vi "SO2 43c Serial Data Recording & DECADEv3.6_test.vi"() -> ()   [LabVIEW 2014]
uses:
  <vilib>/Instr/_visa.llb/VISA Set IO Buffer Mask.ctl
  <vilib>/Platform/TimedLoop/XDataNode/timing_clust.ctl
  <vilib>/Platform/TimedLoop/XDataNode/nitl_modes.ctl
  <vilib>/Platform/TimedLoop/XDataNode/wakeup.ctl
  C:/Program Files (x86)/National Instruments/LabVIEW 2014/examples/Data Communication/Network Streams/Simple Network Streams/support/Network Stream Command.ctl
  <vilib>/Utility/error.llb/whitespace.ctl
  <vilib>/Instr/_visa.llb/VISA Configure Serial Port (Instr).vi
  <vilib>/Utility/tcp.llb/UDP Multicast Write-Only Open.vi
  <vilib>/platform/TimedLoop/XDataNode/XDataNode.xnode
  <vilib>/Platform/TimedLoop/XDataNode/XDNodeRunTimeDep.lvlib
panel:
  out "Default file name":string
  out "Stop File Write":bool
  out "error out 4":errorcluster
  out "Data Array UDP":string[](array[string])
  out "Slope":dbl=0.87463
  out "Offset":dbl
  out "Simulate TWA Conc":dbl
  out "8hr_TWA_limit":i32=490
  out "10mins_STEL_limit":i32=700
  out "Simulate STEL Conc":dbl
  out "Simulate\nconc":bool
  out "q_size 2":i32
  out "8hr_so2_avg 2":dbl=1.0
  out "10min_so2_avg":dbl=1.0
  out "q_size":i32
  in  "Clear Display\nErrors":bool
  in  "dummy2":string="0"
  out "Data Processing":bool
  out "Serial Visa Error":errorcluster
  out "SEPTIC TCP Error Out":errorcluster
  out "TCP packet\nSend to SEPTIC":bool
  in  "Time Stamp\nOffset":u32=1
  out "Data Array TCP":string[](array[string])
  out "UDP packet \nstatus":bool
  out "UDP_Out_Error":errorcluster
  out "FISH TCP Error Out":errorcluster
  out "TCP packet\nSend to FISH":bool
  out "TCP Binary Packet":string
  out "Scan from String Error Counter\nfrom process loop":i32
  out "Read Error Counter\nfrom process loop":i32
  in  "milliseconds to wait":u32=330
  in  "ID":string="«"
  in  "VISA resource name":refnum<visa-resource-name>="ASRL6::INSTR"
  out "Data In Array":string[](array[string])
  out "UDP_ASCII_Out":string
  out "UDP_Pack_num":u32
  out "Flight Number":string
  in  "dummy1":string="00"
  out "Data String":string
  out "Internal packet":string[](array[string])
  out "RAW DATA":string
  in  "stop":bool
  out "Number of Send & Read Error\nfrom Acquire Loop":i32
  out "Command In":string
  # "SO2_conc"
  # "PMT_Volt"
  # "Lamp_Volt"
  # "Lamp_Intensity_Hz"
  # "Internal_Temp_degC"
  # "Reaction_Chamber_Temp_degC"
  # "Reaction_Chamber_Press_mmHg"
  # "Sample_Flow_litre_per_minute"
  # "Flag"
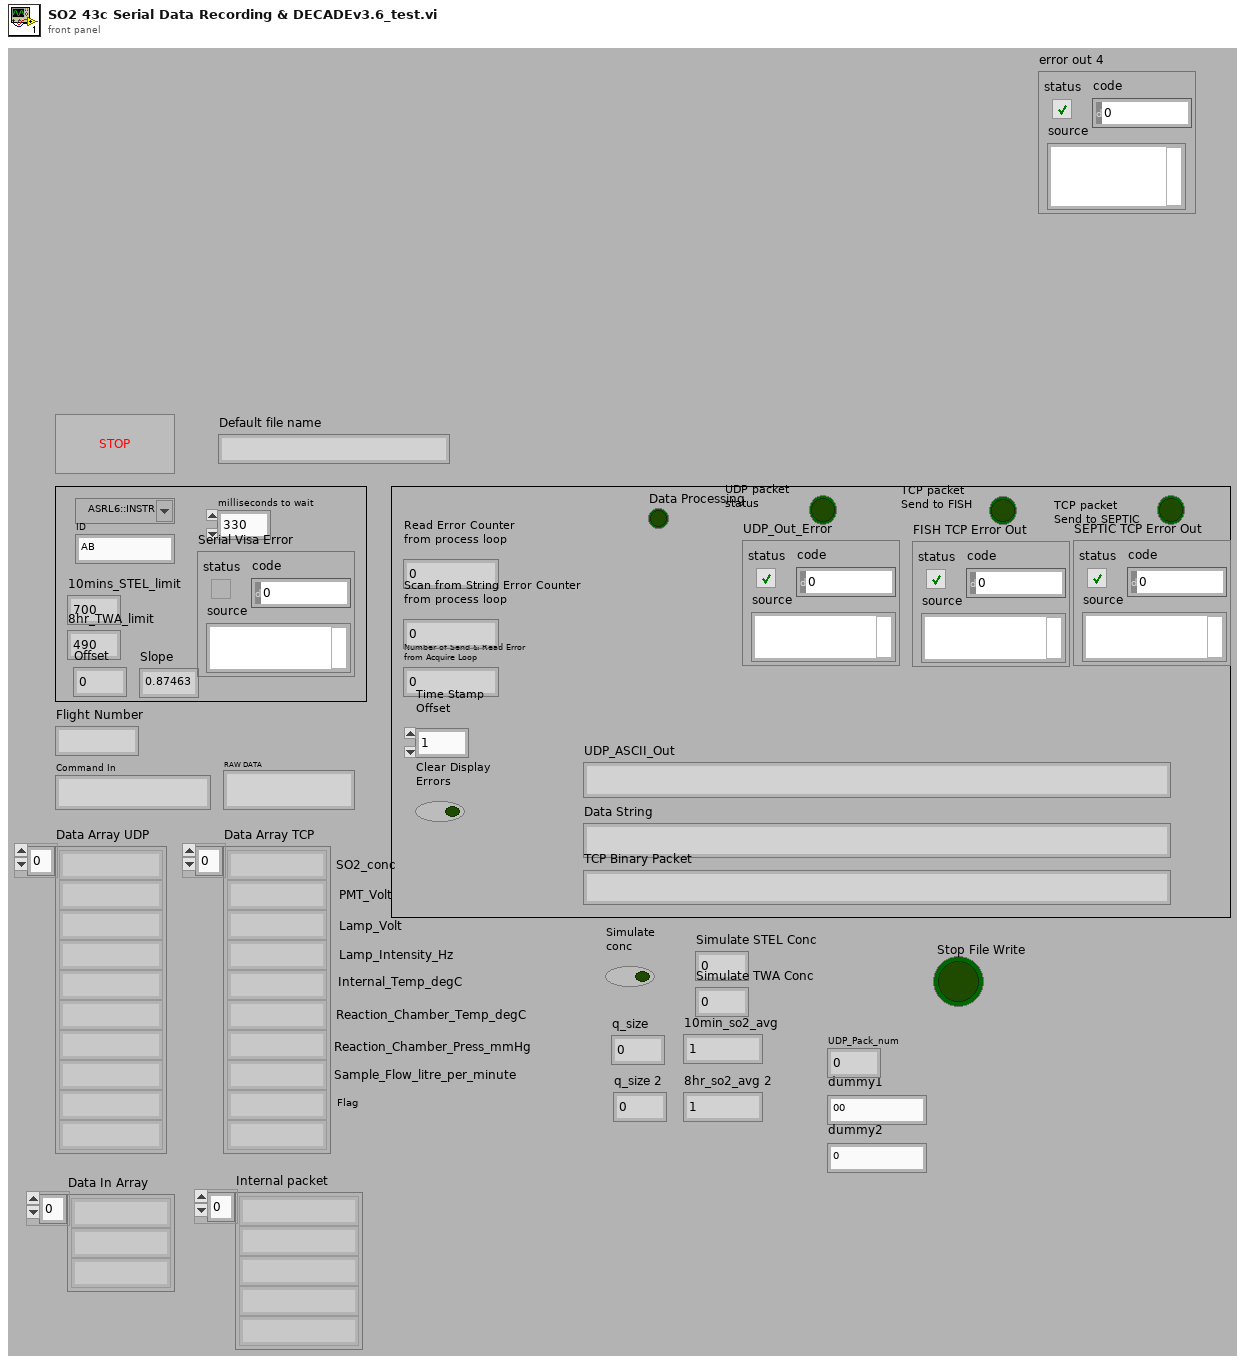
[diagram p1: front panel]
types:
  T1 = typedef "VISA Set IO Buffer Mask.ctl" = u16
  T2 = typedef "Network Stream Command.ctl" = cluster{"Message":string, "Message Data":variant}
  T3 = typedef "XDNodeRunTimeDep.lvlib/timing_clust.ctl" = cluster{"Expected End [f-1]":u64, "Actual End [f-1]":u64, "Finished Late? [f-1]":bool, "Expected End [i-1]":u64, "Actual End [i-1]":u64, "Finished Late? [i-1]":bool, "Expected Start [i]":u64, "Actual Start [i]":u64, "Expected Start [f]":u64, "Actual Start [f]":u64, "Source Name":string, "Structure Name":string, "Period":i64, "Deadline":i64, "Offset":i64, "Start":i64, "Priority":i32, "Timeout":i32, "Mode":T4, "Wakeup Reason":T5, "Error":errorcluster, "Source Type":string, "Secondary Source Type":string, "Global End Time":u64, "Global Start Time":u64, "Frame Duration":u64, "Iteration Duration":u64, "Assigned CPU":i32, "I/O Scan Engine Mode":u32}
  T4 = typedef "XDNodeRunTimeDep.lvlib/nitl_modes.ctl" = enum32{"No Change", "Process missed periods, maintain original phase", "Discard missed periods, maintain original phase", "Process missed periods, ignore original phase", "Discard missed periods, ignore original phase"}
  T5 = typedef "XDNodeRunTimeDep.lvlib/wakeup.ctl" = enum32{"Normal", "Aborted", "Asynchronous wakeup", "Timing source error", "Timed loop error", "Timeout"}
  T6 = enum16{"open", "replace", "create", "open or create", "replace or create", "replace or create with confirmation"}
  T7 = typedef "whitespace.ctl" = u16
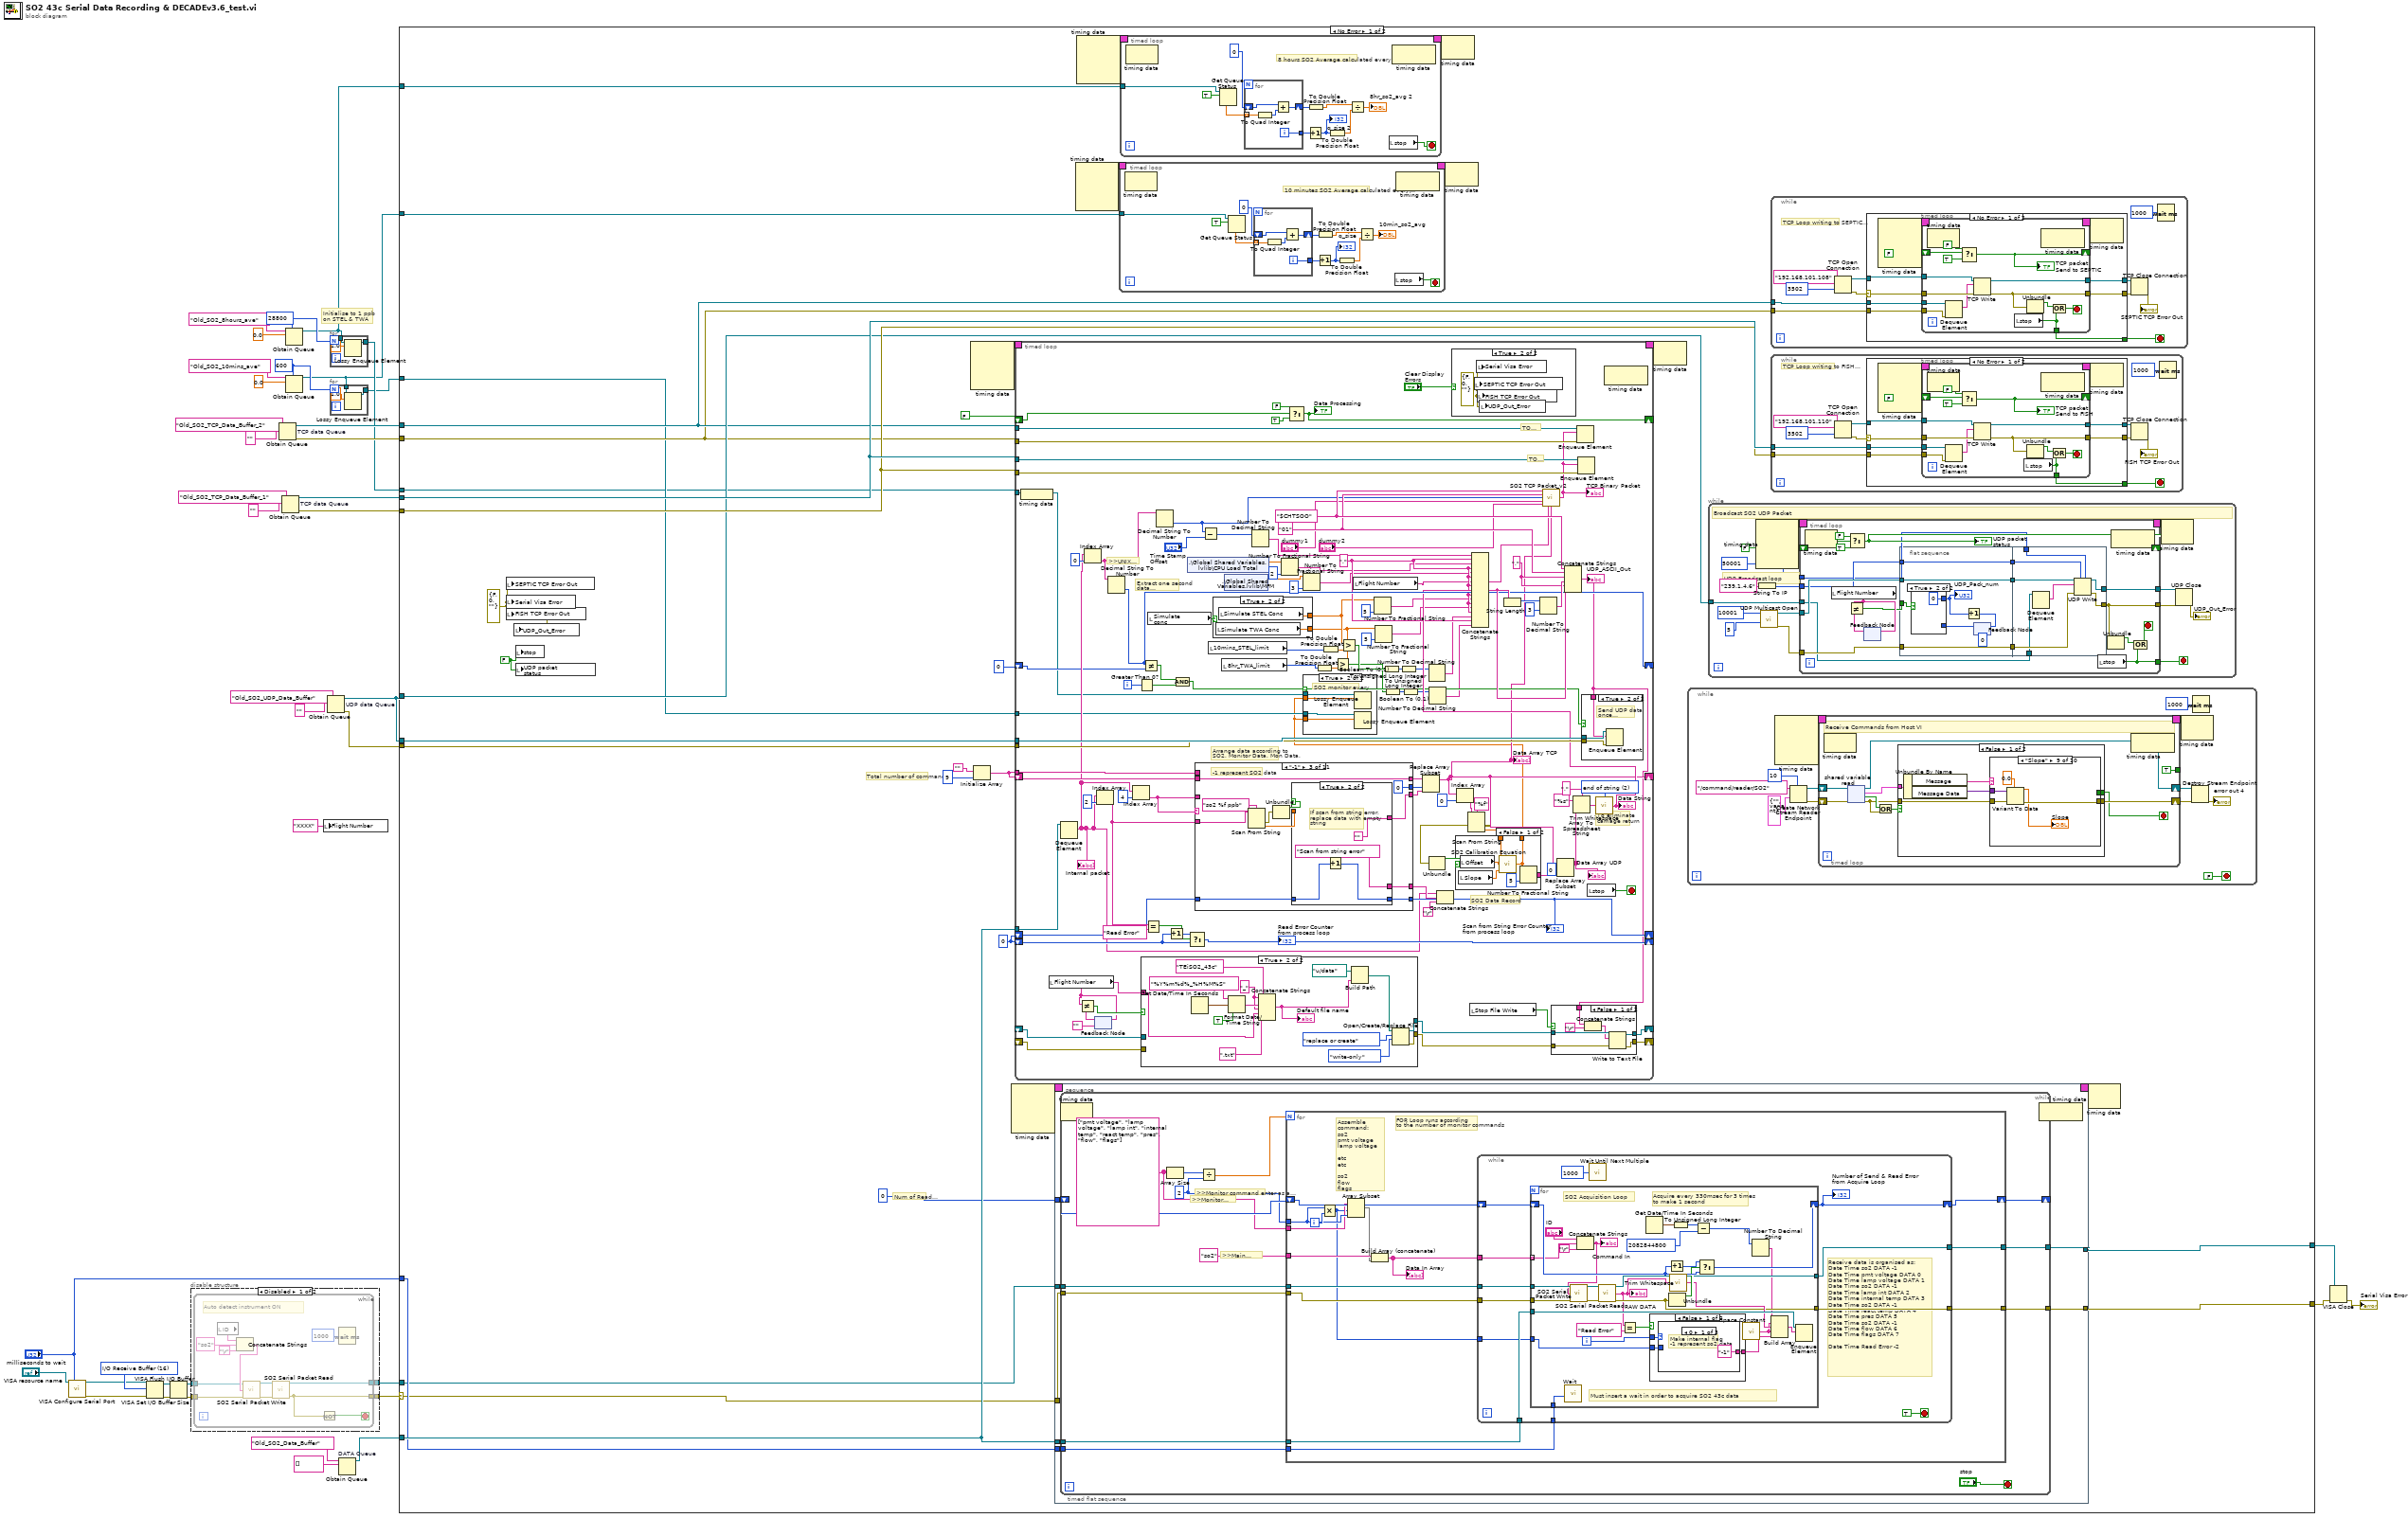
[diagram p0: block diagram]
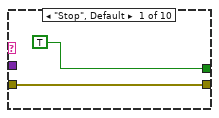
[diagram p3: hidden frame]
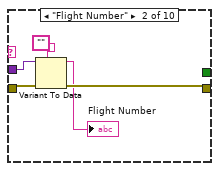
[diagram p4: hidden frame]
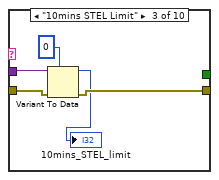
[diagram p5: hidden frame]
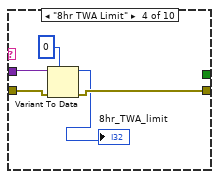
[diagram p6: hidden frame]
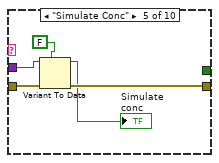
[diagram p7: hidden frame]
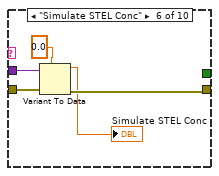
[diagram p8: hidden frame]
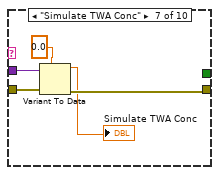
[diagram p9: hidden frame]
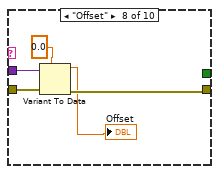
[diagram p10: hidden frame]
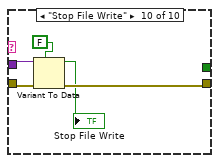
[diagram p11: hidden frame]
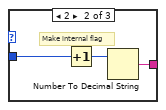
[diagram p13: hidden frame]
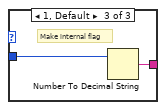
[diagram p14: hidden frame]
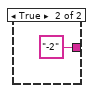
[diagram p15: hidden frame]
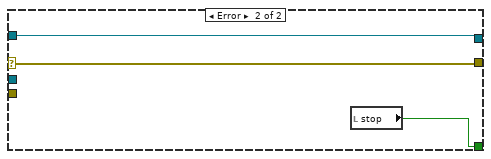
[diagram p16: hidden frame]
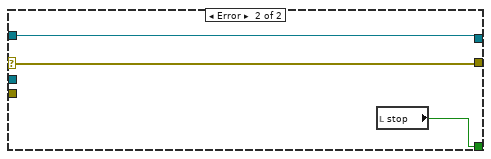
[diagram p18: hidden frame]
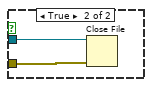
[diagram p20: hidden frame]
diagram:
  w10 = T1 16 items=["I/O Receive Buffer"=16, "I/O Transmit Buffer"=32, "I/O Receive and Transmit Buffer"=48] ("Mask")
  w16 = 28800 ("max queue size (-1, unlimited)")
  w13 = 600 ("max queue size (-1, unlimited)")
  # "Initialise to 1 ppb\non STEL & TWA"
  n1 = call-poly "VISA Configure Serial Port"("VISA resource name"="VISA resource name", "timeout (10sec)"="milliseconds to wait") -> ("VISA resource name out"=w9:refnum<visa-resource-name>, "error out"=w8:errorcluster)  [unwired: 12 in]
  n2 = VISA Set I/O Buffer Size(VISA resource name=w9, mask (16)=w10, error in (no error)=w8) -> (VISA resource name out=w6:refnum<visa-resource-name>, error out=w7:errorcluster)  [unwired: 1 in]
  n3 = VISA Flush I/O Buffer(VISA resource name=w6, error in (no error)=w7) -> (VISA resource name out=w5:refnum<visa-resource-name>, error out=w4:errorcluster)  [unwired: 1 in]
  n4 = disable-structure shown="Disabled" {
    disable-tunnel: w5 -> [w44 _]
    disable-tunnel: w4 -> [w43 _]
    disable-tunnel: [w42 _] -> w3
    disable-tunnel: [w41 _] -> w2
    frame Disabled {
      n5 = while {
        tunnel: w44 -> [w52]
        tunnel: w43 -> [w51]
        tunnel: [w47] -> w42
        tunnel: [w46] -> w41
        stop <- w48 stop-if-true
        # "Auto detect instrument ON"
        n6 = local read "ID"() -> (w55:string)
        n7 = Concatenate Strings(w55, "so2" ("string"), "\r") -> (w53:string)
        n8 = call "SO2 Serial Packet Write.vi"("VISA resource name In"=w52, "Data in"=w53, "error in (no error)"=w51) -> ("VISA resource name Out"=w49:refnum<visa-resource-name>, "error out"=w50:errorcluster)  [unwired: 11 in]
        n9 = call "SO2 Serial Packet Read.vi"("VISA resource In"=w49, "error in"=w50) -> ("VISA resource Out"=w46:refnum<visa-resource-name>, "error out"=w47:errorcluster)  [unwired: 11 in, 1 out]
        n10 = Not(x=w47) -> (.not. x?=w48:bool)
        n11 = Wait (ms)(milliseconds to wait=u32 1000) -> ()  [unwired: 1 out]
      }
    }
    frame Enabled {
    }
  }
  n12 = Obtain Queue "TCP data Queue"(name (unnamed)="Old_SO2_TCP_Data_Buffer_2", element data type="") -> (queue out=w23:refnum<queue>, error out=w22:errorcluster)  [unwired: 3 in, 1 out]
  n13 = Obtain Queue "TCP data Queue"(name (unnamed)="Old_SO2_TCP_Data_Buffer_1", element data type="") -> (queue out=w31:refnum<queue>, error out=w30:errorcluster)  [unwired: 3 in, 1 out]
  n14 = Obtain Queue(max queue size (-1, unlimited)=w16, name (unnamed)="Old_SO2_8hours_ave", element data type=0.0 ("index")) -> (queue out=w15:refnum<queue>)  [unwired: 2 in, 2 out]
  n15 = Obtain Queue(max queue size (-1, unlimited)=w13, name (unnamed)="Old_SO2_10mins_ave", element data type=0.0 ("index")) -> (queue out=w12:refnum<queue>)  [unwired: 2 in, 2 out]
  n16 = local write "Flight Number"("XXXX" ("Flight Number")) -> ()
  n17 = Obtain Queue "UDP data Queue"(name (unnamed)="Old_SO2_UDP_Data_Buffer", element data type="") -> (queue out=w26:refnum<queue>, error out=w27:errorcluster)  [unwired: 3 in, 1 out]
  n18 = for {
    N: w16 -> [_]
    tunnel: w15 -> [w59]
    tunnel: [w58] -> w14
    n19 = Lossy Enqueue Element(queue=w59, element=1.0) -> (queue out=w58:refnum<queue>)  [unwired: 1 in, 3 out]
  }
  n20 = for {
    N: w13 -> [_]
    tunnel: [w62] -> w11
    tunnel: w12 -> [w60]
    n21 = Lossy Enqueue Element(queue=w60, element=1.0) -> (queue out=w62:refnum<queue>)  [unwired: 1 in, 3 out]
  }
  n22 = Obtain Queue "DATA Queue"(name (unnamed)="Old_SO2_Data_Buffer", element data type=string[] []) -> (queue out=w38:refnum<queue>)  [unwired: 3 in, 2 out]
  n23 = case shown="No Error" w3 {
    selector: w3 -> [w65 w822]
    tunnel: [w96 w822] -> w35
    tunnel: [w95 w821] -> w36
    tunnel: w38 -> [w92 _]
    tunnel: w2 -> [w66 w821]
    tunnel: w31 -> [w85 _]
    tunnel: w30 -> [w84 _]
    tunnel: w26 -> [w83 _]
    tunnel: w27 -> [w82 _]
    tunnel: w26 -> [w81 _]
    tunnel: w23 -> [w79 _]
    tunnel: w22 -> [w78 _]
    tunnel: "milliseconds to wait" -> [w77 _]
    tunnel: w12 -> [w74 _]
    tunnel: w15 -> [w73 _]
    tunnel: w11 -> [w72 _]
    tunnel: w14 -> [w71 _]
    frame No Error {
      w75 = errorcluster {"status"=FALSE, "code"=0, "source"=""} ("UDP Error Out")
      w87 = 0
      w86 = FALSE ("stop")
      # "Num of Read Error"
      # "Total number of commands"
      n24 = local write "SEPTIC TCP Error Out"(w75) -> ()
      n25 = local write "Serial Visa Error"(w75) -> ()
      n26 = local write "FISH TCP Error Out"(w75) -> ()
      n27 = local write "UDP_Out_Error"(w75) -> ()
      n28 = local write "stop"(w86) -> ()
      n29 = local write "UDP packet \nstatus"(w86) -> ()
      n30 = node-c288() -> (w94:T3)  [unwired: 4 in]
      n31 = Initialize Array("", 9) -> (w88:string[])
      n32 = node-c288() -> (w64:T3)  [unwired: 4 in]
      n33 = timed-loop {
        timing: w94 -> [_]
        timing-out: [_] -> w93
        tunnel: w92 -> [w568]
        shift-right: [w485] -> _
        shift-left: w88 -> [w558]
        shift-right: [w549] -> _
        shift-left: w87 -> [w546]
        tunnel: w88 -> [w548]
        shift-right: [w544] -> _
        shift-left: w87 -> [w545]
        tunnel: w85 -> [w539]
        tunnel: w84 -> [w538]
        tunnel: w83 -> [w537]
        tunnel: w82 -> [w536]
        shift-right: [w528] -> _
        shift-left: 0 -> [w531]
        tunnel: w79 -> [w527]
        tunnel: w78 -> [w526]
        shift-right: [w517] -> _
        shift-left: FALSE -> [w520]
        tunnel: w72 -> [w511]
        tunnel: w71 -> [w510]
        shift-right: [w470] -> _
        shift-left: _ -> [w467]
        shift-right: [w469] -> _
        shift-left: _ -> [w465]
        i -> [w529]
        stop <- w566 stop-if-true
        w554 = T7 2 items=["both", "start of string", "end of string"] ("location (both)")
        w509 = ","
        w541 = "01"
        w560 = ","
        w542 = "$CHTSOO"
        # "TO SEPTIC"
        # "TO FISH"
        # "Extract one second data\nfor UDP sending"
        # "Arrange data according to\nSO2, Monitor Data, Mon Data,"
        # "To eliminate\ncarriage return"
        # ">>UNIX TIME>>"
        # "SO2 Data Record"
        n34 = node-c288() -> ()  [unwired: 1 in]
        n35 = local read "Flight Number"() -> (w466:string)
        n36 = Dequeue Element(queue=w568) -> (element=w534:string[])  [unwired: 2 in, 3 out]
        "Internal packet" <- w534
        n37 = Index Array(array=w534, index=0) -> (element=w533:string)
        n38 = feedback #1("" ("Flight Number")) -> (w475:string)
        n39 = Not Equal?(x=w466, y=w475) -> (x != y?=w473:bool)
        n40 = feedback-in #1(w466) -> ()
        n41 = Index Array(array=w534, index=2) -> (element=w552:string)
        n42 = Decimal String To Number(string=w533) -> (number=w528:i32)  [unwired: 2 in, 1 out]
        n43 = Index Array(array=w534, index=4) -> (element=w516:string)
        n44 = Greater Than 0?(x=w529) -> (x > 0?=w532:bool)
        n45 = case shown="True" w473 {
          tunnel: [w570 w573] -> w472
          tunnel: [w569 w572] -> w468
          tunnel: w467 -> [w570 _]
          tunnel: w465 -> [w569 _]
          tunnel: w466 -> [_ w571]
          frame False {
          }
          frame True {
            w580 = "_" ("string")
            n46 = Get Date/Time In Seconds() -> (seconds since 1Jan1904=w581:timestamp)
            n47 = Format Date/Time String(time format string (%c)="%Y%m%d%_%H%M%S", seconds (now)=w581, UTC format=TRUE) -> (date/time string=w584:string)
            n48 = Concatenate Strings("TEiSO2_43c" ("string"), w580, w584, w580, w571, ".txt" ("string")) -> (w578:string)
            "Default file name" <- w578
            n49 = Build Path(base path=path "u:/data", name or relative path=w578) -> (appended path=w574:path)
            n50 = Open/Create/Replace File(file path (use dialog)=w574, operation (0:open)=T6."replace or create", access (0:read/write)=enum16{"read/write", "read-only", "write-only"}."write-only") -> (refnum out=w573:refnum<file>, error out=w572:errorcluster)  [unwired: 3 in, 1 out]
          }
        }
        n51 = Not Equal?(x=w528, y=w531) -> (x != y?=w530:bool)
        n52 = Equal?(x=w552, y="Read Error") -> (x = y?=w550:bool)
        n53 = local read "Simulate\nconc"() -> (w479:bool)
        n54 = Decimal String To Number(string=w533) -> (number=w523:i32)  [unwired: 2 in, 1 out]
        n55 = Increment(x=w546) -> (x+1=w547:i32)
        n56 = Compound Arithmetic op=AND(w530, w532) -> (w512:bool)
        n57 = shared-variable ".\\Global Shared Variables.lvlib\\CPU Load Total"() -> (w463:dbl)  [unwired: 1 in, 1 out]
        n58 = Select(t=w547, s=w550, f=w546) -> (s? t:f=w549:i32)
        "Read Error Counter\nfrom process loop" <- w549
        n59 = case shown="\"-1\"" w516 {
          tunnel: w516 -> [w620 _ _ w656 w677 w698 w720 w742 w764 w786 w808]
          tunnel: w558 -> [w621 _ w635 w657 w678 w699 w721 w743 w765 w787 w809]
          tunnel: w552 -> [_ _ w632 w652 w673 w695 w717 w739 w761 w783 w805]
          tunnel: [w621 w624 w635 w657 w678 w699 w721 w743 w765 w787 w809] -> w492
          tunnel: [w618 _ 0 ("index") w654 w675 w696 w718 w740 w762 w784 w806] -> w491
          tunnel: [_ _ w631 w651 w672 w694 w716 w738 w760 w782 w800] -> w557
          tunnel: w548 -> [_ w624 _ _ _ _ _ _ _ _ _]
          tunnel: w545 -> [w616 w623 w628 w648 w669 w689 w712 w733 w756 w777 w799]
          tunnel: [w616 w623 w627 w647 w668 w688 w711 w732 w755 w776 w798] -> w544
          tunnel: ["Internal False Flag Detected" "" w626 w646 w667 w687 w710 w731 w754 w775 w797] -> w543
          frame "False", Default {
            n60 = Decimal String To Number(string=w620) -> (number=w617:i32)  [unwired: 2 in, 1 out]
            n61 = Add(x=w617, y=1) -> (x+y=w618:i32)
          }
          frame "-2" {
            # "Read Error Detected\nMake all data as a space"
          }
          frame "-1" {
            # "-1 represent SO2 data"
            n62 = Scan From String(format string="so2 %f ppb", input string=w632) -> (error out=w630:errorcluster, output 1=w625:dbl)  [unwired: 3 in, 2 out]
            n63 = Unbundle(w630) -> ("status"=w629:bool)  [unwired: 2 out]
            n64 = case shown="True" w629 {
              tunnel: w625 -> [w636 _]
              tunnel: [w640 ""] -> w631
              tunnel: w628 -> [w639 w644]
              tunnel: [w639 w643] -> w627
              tunnel: ["" "Scan from string error"] -> w626
              frame False {
                # "Extract the concentration\nvalue & fixed format"
                n65 = Number To Fractional String(number=w636, precision (6)=i16 5) -> (F-format string=w640:string)  [unwired: 2 in]
              }
              frame True {
                # "If scan from string error,\nreplace data with empty\nstring"
                n66 = Increment(x=w644) -> (x+1=w643:i32)
              }
            }
          }
          frame "0" {
            # "0 represents pmt voltage -0510 volts"
            n67 = Scan From String(format string="pmt voltage %d volts", input string=w652) -> (error out=w650:errorcluster, output 1=w645:i32)  [unwired: 3 in, 2 out]
            n68 = Decimal String To Number(string=w656) -> (number=w655:i32)  [unwired: 2 in, 1 out]
            n69 = Unbundle(w650) -> ("status"=w649:bool)  [unwired: 2 out]
            n70 = case shown="False" w649 {
              tunnel: w645 -> [w661 _]
              tunnel: [w658 w662] -> w651
              tunnel: w648 -> [w660 w665]
              tunnel: [w660 w664] -> w647
              tunnel: ["" "Scan from string error"] -> w646
              tunnel: [w658 w662] -> _
              frame False {
                # "Extract the actual value\n& fixed format"
                n71 = Number To Decimal String(number=w661) -> (decimal integer string=w658:string)  [unwired: 1 in]
              }
              frame True {
                w662 = ""
                # "If scan from string error,\nreplace data with empty\nstring"
                n72 = Increment(x=w665) -> (x+1=w664:i32)
              }
            }
            n73 = Increment(x=w655) -> (x+1=w654:i32)
          }
          frame "1" {
            # "1 represents lamp voltage; lamp voltage 810 volts"
            n74 = Scan From String(format string="lamp voltage %d volts", input string=w673) -> (error out=w671:errorcluster, output 1=w666:i32)  [unwired: 3 in, 2 out]
            n75 = Decimal String To Number(string=w677) -> (number=w676:i32)  [unwired: 2 in, 1 out]
            n76 = Unbundle(w671) -> ("status"=w670:bool)  [unwired: 2 out]
            n77 = case shown="True" w670 {
              tunnel: w666 -> [w682 _]
              tunnel: [w679 w683] -> w672
              tunnel: w669 -> [w681 w686]
              tunnel: [w681 w685] -> w668
              tunnel: ["" "Scan from string error"] -> w667
              tunnel: [w679 w683] -> _
              frame False {
                # "Extract the actual value\n& fixed format"
                n78 = Number To Decimal String(number=w682) -> (decimal integer string=w679:string)  [unwired: 1 in]
              }
              frame True {
                w683 = ""
                # "If scan from string error,\nreplace data with empty\nstring"
                n79 = Increment(x=w686) -> (x+1=w685:i32)
              }
            }
            n80 = Increment(x=w676) -> (x+1=w675:i32)
          }
          frame "2" {
            # "2 represents lamp intensity; lamp int 35867 Hz"
            n81 = Scan From String(format string="lamp int %d Hz", input string=w695) -> (error out=w691:errorcluster, output 1=w692:i32)  [unwired: 3 in, 2 out]
            n82 = Decimal String To Number(string=w698) -> (number=w697:i32)  [unwired: 2 in, 1 out]
            n83 = Unbundle(w691) -> ("status"=w690:bool)  [unwired: 2 out]
            n84 = case shown="True" w690 {
              tunnel: [w700 w705] -> w694
              tunnel: w692 -> [w704 _]
              tunnel: w689 -> [w703 w708]
              tunnel: [w703 w707] -> w688
              tunnel: ["" "Scan from string error"] -> w687
              tunnel: [w700 w705] -> _
              frame False {
                # "Extract the actual value\n& fixed format"
                n85 = Number To Fractional String(number=w704, precision (6)=i16 0) -> (F-format string=w700:string)  [unwired: 2 in]
              }
              frame True {
                w705 = ""
                # "If scan from string error,\nreplace data with empty\nstring"
                n86 = Increment(x=w708) -> (x+1=w707:i32)
              }
            }
            n87 = Increment(x=w697) -> (x+1=w696:i32)
          }
          frame "3" {
            # "3 represents internal temp; internal temp 027.2 deg C, actual 027.2"
            n88 = Scan From String(format string="%[^,], %s %f", input string=w717) -> (error out=w714:errorcluster, output 3=w709:dbl)  [unwired: 7 in, 2 out]
            n89 = Decimal String To Number(string=w720) -> (number=w719:i32)  [unwired: 2 in, 1 out]
            n90 = Unbundle(w714) -> ("status"=w713:bool)  [unwired: 2 out]
            n91 = case shown="True" w713 {
              tunnel: [w722 w727] -> w716
              tunnel: w709 -> [w726 _]
              tunnel: w712 -> [w725 w730]
              tunnel: [w725 w729] -> w711
              tunnel: ["" "Scan from string error"] -> w710
              tunnel: [w722 w727] -> _
              frame False {
                # "Extract the actual value\n& fixed format"
                n92 = Number To Fractional String(number=w726, precision (6)=i16 1) -> (F-format string=w722:string)  [unwired: 2 in]
              }
              frame True {
                w727 = ""
                # "If scan from string error,\nreplace data with empty\nstring"
                n93 = Increment(x=w730) -> (x+1=w729:i32)
              }
            }
            n94 = Increment(x=w719) -> (x+1=w718:i32)
          }
          frame "4" {
            # "4 represents react temp; react temp 045.2 deg C"
            n95 = Scan From String(format string="react temp %f deg C", input string=w739) -> (error out=w735:errorcluster, output 1=w736:dbl)  [unwired: 3 in, 2 out]
            n96 = Decimal String To Number(string=w742) -> (number=w741:i32)  [unwired: 2 in, 1 out]
            n97 = Unbundle(w735) -> ("status"=w734:bool)  [unwired: 2 out]
            n98 = case shown="False" w734 {
              tunnel: [w744 w749] -> w738
              tunnel: w736 -> [w748 _]
              tunnel: w733 -> [w747 w752]
              tunnel: [w747 w751] -> w732
              tunnel: ["" "Scan from string error"] -> w731
              tunnel: [w744 w749] -> _
              frame False {
                # "Extract the actual value\n& fixed format"
                n99 = Number To Fractional String(number=w748, precision (6)=i16 1) -> (F-format string=w744:string)  [unwired: 2 in]
              }
              frame True {
                w749 = ""
                # "If scan from string error,\nreplace data with empty\nstring"
                n100 = Increment(x=w752) -> (x+1=w751:i32)
              }
            }
            n101 = Increment(x=w741) -> (x+1=w740:i32)
          }
          frame "5" {
            # "5 represents chamber pressure; pres 760.0 mm Hg, actual 753.4"
            n102 = Scan From String(format string="%[^,], %s %f", input string=w761) -> (error out=w758:errorcluster, output 3=w753:dbl)  [unwired: 7 in, 2 out]
            n103 = Decimal String To Number(string=w764) -> (number=w763:i32)  [unwired: 2 in, 1 out]
            n104 = Unbundle(w758) -> ("status"=w757:bool)  [unwired: 2 out]
            n105 = case shown="False" w757 {
              tunnel: [w766 w771] -> w760
              tunnel: w753 -> [w770 _]
              tunnel: w756 -> [w769 w774]
              tunnel: [w769 w773] -> w755
              tunnel: ["" "Scan from string error"] -> w754
              tunnel: [w766 w771] -> _
              frame False {
                # "Extract the actual value\n& fixed format"
                n106 = Number To Fractional String(number=w770, precision (6)=i16 1) -> (F-format string=w766:string)  [unwired: 2 in]
              }
              frame True {
                w771 = ""
                # "If scan from string error,\nreplace data with empty\nstring"
                n107 = Increment(x=w774) -> (x+1=w773:i32)
              }
            }
            n108 = Increment(x=w763) -> (x+1=w762:i32)
          }
          frame "6" {
            # "6 represents flow data; flow 0.503 l/m"
            n109 = Scan From String(format string="flow %f l/m", input string=w783) -> (error out=w779:errorcluster, output 1=w780:dbl)  [unwired: 3 in, 2 out]
            n110 = Decimal String To Number(string=w786) -> (number=w785:i32)  [unwired: 2 in, 1 out]
            n111 = Unbundle(w779) -> ("status"=w778:bool)  [unwired: 2 out]
            n112 = case shown="True" w778 {
              tunnel: [w792 ""] -> w782
              tunnel: w780 -> [w791 _]
              tunnel: w777 -> [w790 w795]
              tunnel: [w790 w794] -> w776
              tunnel: ["" "Scan from string error"] -> w775
              frame False {
                # "Extract the actual value\n& fixed format"
                n113 = Number To Fractional String(number=w791, precision (6)=i16 3) -> (F-format string=w792:string)  [unwired: 2 in]
              }
              frame True {
                # "If scan from string error,\nreplace data with empty\nstring"
                n114 = Increment(x=w795) -> (x+1=w794:i32)
              }
            }
            n115 = Increment(x=w785) -> (x+1=w784:i32)
          }
          frame "7" {
            # "7 represents flags data; flags 1c100000"
            n116 = Scan From String(format string="flags %s", input string=w805) -> (error out=w803:errorcluster, output 1=w801:string)  [unwired: 3 in, 2 out]
            n117 = Decimal String To Number(string=w808) -> (number=w807:i32)  [unwired: 2 in, 1 out]
            n118 = Unbundle(w803) -> ("status"=w802:bool)  [unwired: 2 out]
            n119 = case shown="False" w802 {
              tunnel: w801 -> [w812 _]
              tunnel: [w812 ""] -> w800
              tunnel: w799 -> [w811 w815]
              tunnel: [w811 w814] -> w798
              tunnel: ["" "Scan from string error"] -> w797
              frame False {
                # "Extract the actual value\n& fixed format"
              }
              frame True {
                # "If scan from string error,\nreplace data with empty\nstring"
                n120 = Increment(x=w815) -> (x+1=w814:i32)
              }
            }
            n121 = Increment(x=w807) -> (x+1=w806:i32)
          }
        }
        "Scan from String Error Counter\nfrom process loop" <- w544
        n122 = Subtract(x=w523, y="Time Stamp\nOffset") -> (x-y=w524:u32)
        n123 = local read "10mins_STEL_limit"() -> (w477:i32)
        n124 = case shown="True" w479 {
          tunnel: [w604 w606] -> w505
          tunnel: [w603 w605] -> w503
          frame False {
            n125 = local read "10min_so2_avg"() -> (w604:dbl)
            n126 = local read "8hr_so2_avg 2"() -> (w603:dbl)
          }
          frame True {
            n127 = local read "Simulate TWA Conc"() -> (w605:dbl)
            n128 = local read "Simulate STEL Conc"() -> (w606:dbl)
          }
        }
        n129 = local read "8hr_TWA_limit"() -> (w476:i32)
        n130 = shared-variable ".\\Global Shared Variables.lvlib\\MFM"() -> (w461:dbl)  [unwired: 1 in, 1 out]
        n131 = Number To Decimal String(number=w524) -> (decimal integer string=w521:string)  [unwired: 1 in]
        n132 = Number To Fractional String(number=w463, precision (6)=i16 2) -> (F-format string=w459:string)  [unwired: 2 in]
        n133 = Select(t=FALSE, s=w520, f=TRUE) -> (s? t:f=w517:bool)
        "Data Processing" <- w517
        n134 = Number To Fractional String(number=w461, precision (6)=i16 3) -> (F-format string=w458:string)  [unwired: 2 in]
        n135 = To Double Precision Float(number=w476) -> (double precision float=w506:dbl)
        n136 = To Double Precision Float(number=w477) -> (double precision float=w507:dbl)
        n137 = Greater?(x=w503, y=w506) -> (0:w496:bool)
        n138 = Greater?(x=w505, y=w507) -> (0:w498:bool)
        n139 = local read "Flight Number"() -> (w478:string)
        n140 = Number To Fractional String(number=w505, precision (6)=i16 5) -> (F-format string=w502:string)  [unwired: 2 in]
        n141 = Number To Fractional String(number=w503, precision (6)=i16 5) -> (F-format string=w501:string)  [unwired: 2 in]
        n142 = Boolean To (0,1)(Boolean=w498) -> (0, 1=w500:i16)
        n143 = Boolean To (0,1)(Boolean=w496) -> (0, 1=w499:i16)
        n144 = To Unsigned Long Integer(number=w500) -> (unsigned 32bit integer=w494:u32)
        n145 = To Unsigned Long Integer(number=w499) -> (unsigned 32bit integer=w493:u32)
        n146 = Replace Array Subset(array=w492, new element=w557, index=w491) -> (w485:string[])
        "Data Array TCP" <- w485
        n147 = Number To Decimal String(number=w494) -> (decimal integer string=w497:string)  [unwired: 1 in]
        n148 = Number To Decimal String(number=w493) -> (decimal integer string=w495:string)  [unwired: 1 in]
        n149 = Concatenate Strings(w534, w543, "\r") -> ()  [unwired: 1 out]
        n150 = case shown="True" "Clear Display\nErrors" {
          frame False {
          }
          frame True {
            w611 = errorcluster {"status"=FALSE, "code"=0, "source"=""} ("UDP Error Out")
            n151 = local write "SEPTIC TCP Error Out"(w611) -> ()
            n152 = local write "Serial Visa Error"(w611) -> ()
            n153 = local write "FISH TCP Error Out"(w611) -> ()
            n154 = local write "UDP_Out_Error"(w611) -> ()
          }
        }
        n155 = Index Array(array=w485, index=0) -> (element=w489:string)
        n156 = Scan From String(format string="%f", input string=w489) -> (error out=w481:errorcluster, output 1=w487:dbl)  [unwired: 3 in, 2 out]
        n157 = Unbundle(w481) -> ("status"=w480:bool)  [unwired: 2 out]
        n158 = case shown="False" w480 {
          tunnel: w487 -> [w599 _]
          tunnel: [w598 ""] -> w486
          tunnel: [w597 0.0 ("Output")] -> w482
          frame False {
            n159 = local read "Slope"() -> (w595:dbl)
            n160 = local read "Offset"() -> (w596:dbl)
            n161 = call "SO2 Calibration Equation.vi"("Input"=w599, "Offset"=w596, "Slope"=w595) -> ("Output"=w597:dbl)  [unwired: 12 in]
            n162 = Number To Fractional String(number=w597, precision (6)=i16 5) -> (F-format string=w598:string)  [unwired: 2 in]
          }
          frame True {
          }
        }
        n163 = case shown="True" w512 {
          tunnel: w511 -> [_ w610]
          tunnel: w482 -> [_ w607]
          tunnel: w482 -> [_ w609]
          tunnel: w510 -> [_ w608]
          frame False {
          }
          frame True {
            # "SO2 monitor every second"
            n164 = Lossy Enqueue Element(queue=w610, element=w607) -> ()  [unwired: 1 in, 4 out]
            n165 = Lossy Enqueue Element(queue=w608, element=w609) -> ()  [unwired: 1 in, 4 out]
          }
        }
        n166 = local read "Stop File Write"() -> (w471:bool)
        n167 = call "SO2 TCP Packet_v2.vi"("ID"=w542, "Version"=w541, "utc_time"=w523, "dummy1"="dummy1", "dummy2"="dummy2", "Flight Number"=w478, "Data Array"=w485) -> ("TCP Binary Packet"=w525:string)  [unwired: 8 in]
        "TCP Binary Packet" <- w525
        n168 = Replace Array Subset(array=w485, new element=w486, index=0) -> (w484:string[])
        "Data Array UDP" <- w484
        n169 = Array To Spreadsheet String(delimiter (Tab)=",", array=w484, 3:"%s" ("format string")) -> (spreadsheet string=w553:string)
        n170 = Enqueue Element(queue=w527, element=w525, error in (no error)=w526) -> ()  [unwired: 1 in, 3 out]
        n171 = Enqueue Element(queue=w539, element=w525, error in (no error)=w538) -> ()  [unwired: 1 in, 3 out]
        n172 = local read "stop"() -> (w566:bool)
        n173 = call <vilib>:"Trim Whitespace.vi"("string"=w553, "location (both)"=w554) -> ("trimmed string"=w515:string)
        "Data String" <- w515
        n174 = Concatenate Strings(w521, w509, w459, w509, w458, w509, w478, w509, w515, w509, w502, w509, w501, w509, w497, w509, w495) -> (w559:string)
        n175 = String Length(string=w559) -> (length=w563:i32)
        n176 = Number To Decimal String(number=w563, width (-)=i16 3) -> (decimal integer string=w561:string)
        n177 = Concatenate Strings(w542, w541, w560, w561, w560, w559) -> (w464:string)
        "UDP_ASCII_Out" <- w464
        n178 = case shown="False" w471 {
          tunnel: w464 -> [w590 _]
          tunnel: w472 -> [w592 w594]
          tunnel: w468 -> [w591 w593]
          tunnel: [w587 _] -> w470
          tunnel: [w586 _] -> w469
          frame False {
            n179 = Concatenate Strings(w590, "\r") -> (w588:string)
            n180 = Write to Text File(file (use dialog)=w592, text=w588, error in=w591) -> (refnum out=w587:refnum<file>, error out=w586:errorcluster)  [unwired: 2 out]
          }
          frame True {
            n181 = Close File(refnum=w594, error in=w593) -> ()  [unwired: 2 out]
          }
        }
        n182 = case shown="True" w512 {
          tunnel: w537 -> [_ w614]
          tunnel: w536 -> [_ w613]
          tunnel: w464 -> [_ w612]
          frame False {
          }
          frame True {
            # "Send UDP data once\na second"
            n183 = Enqueue Element(queue=w614, element=w612, error in (no error)=w613) -> ()  [unwired: 1 in, 3 out]
          }
        }
        n184 = node-c288() -> ()  [unwired: 1 in, 1 out]
      }
      n185 = timed-sequence {
        timing: w64 -> [_]
        timing-out: [_] -> w63
        tunnel: [w184] -> w96
        tunnel: [w183] -> w95
        tunnel: w92 -> [w182]
        tunnel: 0 -> [w181]
        tunnel: w77 -> [w180]
        tunnel: w66 -> [w179]
        tunnel: w65 -> [w178]
        n186 = timed-flat-sequence {
          tunnel: [w191] -> w184
          tunnel: [w190] -> w183
          tunnel: w182 -> [w189]
          tunnel: w181 -> [w188]
          tunnel: w180 -> [w187]
          tunnel: w179 -> [w186]
          tunnel: w178 -> [w185]
          n187 = node-c288() -> ()  [unwired: 1 in, 1 out]
          n188 = while {
            tunnel: [w194] -> w191
            tunnel: w186 -> [w205]
            tunnel: w185 -> [w204]
            tunnel: [w203] -> w190
            tunnel: w189 -> [w202]
            shift-right: [w200] -> _
            shift-left: w188 -> [w201]
            tunnel: w187 -> [w192]
            stop <- "stop" stop-if-true
            w195 = 2
            w197 = string[] ["pmt voltage", "lamp voltage", "lamp int", "internal temp", "react temp", "pres", "flow", "flags"]
            # ">>Monitor command enter as a pair>>"
            # ">>Main commands>>"
            # ">>Monitor Command>>"
            n189 = Array Size(array=w197) -> (size(s)=w198:i32)
            n190 = Divide(x=w198, y=w195) -> (x/y=w196:dbl)
            n191 = for {
              N: w196 -> [_]
              tunnel: w205 -> [w213]
              tunnel: w204 -> [w212]
              tunnel: [w220] -> w194
              shift-right: [w218] -> w200
              shift-left: w201 -> [w219]
              tunnel: [w217] -> w203
              tunnel: w202 -> [w216]
              tunnel: w197 -> [w209]
              tunnel: "so2" -> [w214]
              tunnel: w195 -> [w210]
              tunnel: w192 -> [w206]
              i -> [w211]
              # "FOR Loop runs according\nto the number of monitor commands"
              # "Assemble command:\nso2\npmt voltage\nlamp voltage\n\netc\netc\n\nso2\nflow\nflags"
              n192 = Multiply(x=w210, y=w211) -> (x*y=w207:i32)
              n193 = Array Subset(array=w209, index=w207, length=w210) -> (w208:string[])
              n194 = Build Array (concatenate)(w214, w208) -> (w215:string[])
              "Data In Array" <- w215
              n195 = while {
                tunnel: [w232] -> w220
                tunnel: w215 -> [w230]
                tunnel: [w228] -> w217
                tunnel: w216 -> [w227]
                tunnel: w212 -> [w226]
                tunnel: w213 -> [w225]
                tunnel: w207 -> [w224]
                shift-right: [w229] -> w218
                shift-left: w219 -> [w231]
                tunnel: w206 -> [w221]
                stop <- TRUE stop-if-true
                # "Receive data is organised as:\nDate Time so2 DATA -1\nDate Time pmt voltage DATA 0\nDate Time lamp voltage DATA 1\nDate Time so2 DATA -1\nDate Time lamp int DATA 2\nDate Time internal temp DATA 3\nDate Time so2 DATA -1\nDate Time react temp DATA 4\nDate Time pres DATA 5\nDate Time so2 DATA -1\nDate Time flow DATA 6\nDate Time flags DATA 7\n\nDate Time Read Error -2"
                n196 = for {
                  tunnel: w226 -> [w249]
                  tunnel: [w250] -> w232
                  tunnel: w230 -> [w247] mode=indexing
                  tunnel: [w251] -> w228
                  tunnel: w227 -> [w257]
                  tunnel: w225 -> [w252]
                  tunnel: w224 -> [w246]
                  shift-right: [w261] -> w229
                  shift-left: w231 -> [w262]
                  tunnel: w221 -> [w235]
                  i -> [w239]
                  # "Must insert a wait in order to acquire SO2 43c data"
                  # "Acquire every 330msec for 3 times\nto make 1 second"
                  # "SO2 Acquisition Loop"
                  n197 = call "Wait"("Count(mSec)"=w235) -> ()  [unwired: 1 out]
                  n198 = Concatenate Strings("ID", w247, "\r") -> (w245:string)
                  "Command In" <- w245
                  n199 = call "SO2 Serial Packet Write.vi"("VISA resource name In"=w252, "Data in"=w245, "error in (no error)"=w249) -> ("VISA resource name Out"=w254:refnum<visa-resource-name>, "error out"=w253:errorcluster)  [unwired: 11 in]
                  n200 = call "SO2 Serial Packet Read.vi"("VISA resource In"=w254, "error in"=w253) -> ("VISA resource Out"=w251:refnum<visa-resource-name>, "Data Out"=w242:string, "error out"=w250:errorcluster)  [unwired: 11 in]
                  "RAW DATA" <- w242
                  n201 = Equal?(x=w242, y="Read Error") -> (x = y?=w240:bool)
                  n202 = Get Date/Time In Seconds() -> (seconds since 1Jan1904=w234:timestamp)
                  n203 = case shown="False" w240 {
                    tunnel: [w265 "-2"] -> w255
                    tunnel: w239 -> [w264 _]
                    tunnel: w246 -> [w263 _]
                    frame False {
                      n204 = case shown="0" w264 {
                        tunnel: ["-1" w269 w271] -> w265
                        tunnel: w263 -> [_ w267 w270]
                        frame 0 {
                          # "Make internal flag\n-1 represent so2 data"
                        }
                        frame 2 {
                          # "Make internal flag"
                          n205 = Increment(x=w267) -> (x+1=w268:i32)
                          n206 = Number To Decimal String(number=w268) -> (decimal integer string=w269:string)  [unwired: 1 in]
                        }
                        frame 1, Default {
                          # "Make internal flag"
                          n207 = Number To Decimal String(number=w270) -> (decimal integer string=w271:string)  [unwired: 1 in]
                        }
                      }
                    }
                    frame True {
                    }
                  }
                  n208 = Increment(x=w262) -> (x+1=w258:i32)
                  n209 = Unbundle(w250) -> ("status"=w259:bool)  [unwired: 2 out]
                  n210 = call <vilib>:"Trim Whitespace.vi"("string"=w242) -> ("trimmed string"=w256:string)  [unwired: 1 in]
                  n211 = To Unsigned Long Integer(number=w234) -> (unsigned 32bit integer=w238:u32)
                  n212 = Subtract(x=w238, y=u32 2082844800) -> (x-y=w233:u32)
                  n213 = Select(t=w258, s=w259, f=w262) -> (s? t:f=w261:i32)
                  n214 = call <vilib>:"Space Constant.vi"() -> ("String"=w243:string)
                  n215 = Number To Decimal String(number=w233) -> (decimal integer string=w236:string)  [unwired: 1 in]
                  n216 = Build Array(w236, w243, w256, w243, w255) -> (w244:string[])
                  n217 = Enqueue Element(queue=w257, element=w244) -> ()  [unwired: 2 in, 3 out]
                }
                "Number of Send & Read Error\nfrom Acquire Loop" <- w229
                n218 = call "Wait Until Next Multiple"("Count(mSec)"=u32 1000) -> ()  [unwired: 1 out]
              }
            }
          }
          n219 = node-c288() -> ()  [unwired: 1 in, 1 out]
        }
      }
      n220 = node-c288() -> (w68:T3)  [unwired: 4 in]
      n221 = node-c288() -> (w70:T3)  [unwired: 4 in]
      n222 = timed-loop {
        tunnel: w74 -> [w286]
        timing: w68 -> [_]
        timing-out: [_] -> w67
        stop <- w287 stop-if-true
        # "10 minutes SO2 Average calculated every second"
        n223 = node-c288() -> ()  [unwired: 1 in, 1 out]
        n224 = Get Queue Status(queue=w286, return elements? (F)=TRUE) -> (elements=w277:dbl[])  [unwired: 1 in, 7 out]
        n225 = for {
          tunnel: w277 -> [w290] mode=indexing
          tunnel: [w294] -> w283
          shift-right: [w293] -> w281
          shift-left: i64 0 -> [w292]
          i -> [w294]
          n226 = To Quad Integer(1:w290) -> (0:w291:i64)
          n227 = Add(x=w292, y=w291) -> (x+y=w293:i64)
        }
        n228 = Increment(x=w283) -> (x+1=w278:i32)
        "q_size" <- w278
        n229 = To Double Precision Float(number=w281) -> (double precision float=w279:dbl)
        n230 = To Double Precision Float(number=w278) -> (double precision float=w280:dbl)
        n231 = Divide(x=w279, y=w280) -> (x/y=→"10min_so2_avg":dbl)
        n232 = local read "stop"() -> (w287:bool)
        n233 = node-c288() -> ()  [unwired: 1 in, 1 out]
      }
      n234 = timed-loop {
        tunnel: w73 -> [w306]
        timing: w70 -> [_]
        timing-out: [_] -> w69
        stop <- w307 stop-if-true
        # "8 hours SO2 Average calculated every second"
        n235 = node-c288() -> ()  [unwired: 1 in, 1 out]
        n236 = Get Queue Status(queue=w306, return elements? (F)=TRUE) -> (elements=w303:dbl[])  [unwired: 1 in, 7 out]
        n237 = for {
          tunnel: w303 -> [w310] mode=indexing
          tunnel: [w314] -> w302
          shift-right: [w313] -> w300
          shift-left: i64 0 -> [w312]
          i -> [w314]
          n238 = To Quad Integer(1:w310) -> (0:w311:i64)
          n239 = Add(x=w312, y=w311) -> (x+y=w313:i64)
        }
        n240 = Increment(x=w302) -> (x+1=w297:i32)
        "q_size 2" <- w297
        n241 = To Double Precision Float(number=w300) -> (double precision float=w298:dbl)
        n242 = To Double Precision Float(number=w297) -> (double precision float=w299:dbl)
        n243 = Divide(x=w298, y=w299) -> (x/y=→"8hr_so2_avg 2":dbl)
        n244 = local read "stop"() -> (w307:bool)
        n245 = node-c288() -> ()  [unwired: 1 in, 1 out]
      }
      n246 = node-c288(w69) -> ()  [unwired: 1 out]
      n247 = node-c288(w67) -> ()  [unwired: 1 out]
      n248 = node-c288(w93) -> ()  [unwired: 1 out]
      n249 = while {
        stop <- FALSE stop-if-true
        n250 = node-c288() -> (w98:T3)  [unwired: 4 in]
        n251 = Create Network Stream Reader Endpoint(7:10 ("reader buffer size"), 9:T2 {"Message"="", "Message Data"=variant} ("Message Cluster"), 11:"/command/reader/SO2" ("reader url")) -> (0:w104:errorcluster, 3:w105:refnum<k21>)  [unwired: 4 in]
        n252 = timed-loop "Host->Target Command Reader" {
          shift-right: [w115] -> w102
          shift-left: w104 -> [w118]
          shift-right: [w116] -> w101
          shift-left: w105 -> [w117]
          tunnel: [TRUE] -> _
          timing: w98 -> [_]
          timing-out: [_] -> w97
          stop <- w109 stop-if-true
          # "Receive Commands from Host VI"
          n253 = node-c288() -> ()  [unwired: 1 in, 1 out]
          n254 = shared-variable-read(w117, w118) -> (w116:refnum<k21>, w111:errorcluster, w113:bool, w114:T2)  [unwired: 1 in]
          n255 = Or(x=w113, y=w111) -> (x .or. y?=w112:bool)
          n256 = case shown="False" w112 {
            selector: w112 -> [_ w174]
            tunnel: w111 -> [w126 w175]
            tunnel: [w125 w175] -> w115
            tunnel: w114 -> [w123 _]
            tunnel: [w124 w174] -> w109
            frame False {
              n257 = Unbundle By Name(w123) -> ("Message"=w122:string, "Message Data"=w121:variant)
              n258 = case shown="\"Slope\"" w122 {
                tunnel: w126 -> [w128 w133 w138 w143 w148 w152 w157 w162 w167 w173]
                tunnel: [w128 w130 w136 w141 w147 w150 w155 w160 w165 w170] -> w125
                tunnel: w121 -> [_ w132 w137 w142 w146 w153 w158 w163 w168 w172]
                tunnel: [TRUE _ _ _ _ _ _ _ _ _] -> w124
                frame "Stop", Default {
                }
                frame "Flight Number" {
                  n259 = Variant To Data(error in=w133, type="", Variant=w132) -> (data=→"Flight Number":string, error out=w130:errorcluster)
                }
                frame "10mins STEL Limit" {
                  n260 = Variant To Data(error in=w138, type=0, Variant=w137) -> (data=→"10mins_STEL_limit":i32, error out=w136:errorcluster)
                }
                frame "8hr TWA Limit" {
                  n261 = Variant To Data(error in=w143, type=0, Variant=w142) -> (data=→"8hr_TWA_limit":i32, error out=w141:errorcluster)
                }
                frame "Simulate Conc" {
                  n262 = Variant To Data(error in=w148, type=FALSE, Variant=w146) -> (data=→"Simulate\nconc":bool, error out=w147:errorcluster)
                }
                frame "Simulate STEL Conc" {
                  n263 = Variant To Data(error in=w152, type=0.0, Variant=w153) -> (data=→"Simulate STEL Conc":dbl, error out=w150:errorcluster)
                }
                frame "Simulate TWA Conc" {
                  n264 = Variant To Data(error in=w157, type=0.0, Variant=w158) -> (data=→"Simulate TWA Conc":dbl, error out=w155:errorcluster)
                }
                frame "Offset" {
                  n265 = Variant To Data(error in=w162, type=0.0, Variant=w163) -> (data=→"Offset":dbl, error out=w160:errorcluster)
                }
                frame "Slope" {
                  n266 = Variant To Data(error in=w167, type=0.0, Variant=w168) -> (data=→"Slope":dbl, error out=w165:errorcluster)
                }
                frame "Stop File Write" {
                  n267 = Variant To Data(error in=w173, type=FALSE, Variant=w172) -> (data=→"Stop File Write":bool, error out=w170:errorcluster)
                }
              }
            }
            frame True {
            }
          }
          n268 = node-c288() -> ()  [unwired: 1 in, 1 out]
        }
        n269 = node-c288(w97) -> ()  [unwired: 1 out]
        n270 = Destroy Stream Endpoint(8:w102, 11:w101) -> (0:→"error out 4":errorcluster)
        n271 = Wait (ms)(milliseconds to wait=u32 1000) -> ()  [unwired: 1 out]
      }
      n272 = while {
        tunnel: w81 -> [w359]
        stop <- w360 stop-if-true
        # "UDP Broadcast loop"
        # "Broadcast SO2 UDP Packet"
        n273 = node-c288() -> (w362:T3)  [unwired: 4 in]
        n274 = String To IP(1:"239.1.4.6" ("name")) -> (0:w364:u32)
        n275 = call-poly <vilib>:"UDP Multicast Open.vi"("time-to-live (1)"=u16 5, "port"=u16 10001) -> ("error out"=w372:errorcluster, "connection ID"=w373:refnum<k16>)  [unwired: 8 in]
        n276 = timed-loop {
          tunnel: w373 -> [w393]
          tunnel: w372 -> [w392]
          tunnel: [w379] -> w368
          shift-right: [w382] -> _
          shift-left: FALSE -> [w385]
          tunnel: [w377] -> w366
          tunnel: w364 -> [w381]
          tunnel: u16 50001 ("port or service name") -> [w380]
          timing: w362 -> [_]
          timing-out: [_] -> w361
          tunnel: [w375] -> w360
          tunnel: w359 -> [w374]
          stop <- w376 stop-if-true
          n277 = node-c288() -> ()  [unwired: 1 in, 1 out]
          n278 = local read "Flight Number"() -> (w388:string)
          n279 = Select(t=FALSE, s=w385, f=TRUE) -> (s? t:f=w382:bool)
          "UDP packet \nstatus" <- w382
          n280 = feedback-in #2(w388) -> ()
          n281 = feedback #2() -> (w387:string)  [unwired: 1 in]
          n282 = Not Equal?(x=w388, y=w387) -> (x != y?=w386:bool)
          n283 = flat-sequence {
            tunnel: w381 -> [w401]
            tunnel: w392 -> [w402]
            tunnel: w393 -> [w403]
            tunnel: [w403] -> w391
            tunnel: [w402] -> w390
            tunnel: [w401] -> w389
            tunnel: w386 -> [w400]
            tunnel: w380 -> [w413]
            tunnel: w391 -> [w412]
            tunnel: w390 -> [w411]
            tunnel: w389 -> [w410]
            tunnel: [w409] -> w379
            tunnel: [w408] -> w377
            tunnel: w374 -> [w407]
            frame #0 {
              n284 = feedback #3(u32 0) -> (w397:u32)
              n285 = case shown="True" w400 {
                tunnel: w397 -> [w404 _]
                tunnel: [w404 u32 0] -> w396
                frame False {
                }
                frame True {
                }
              }
              "UDP_Pack_num" <- w396
              n286 = Increment(x=w396) -> (x+1=w398:u32)
              n287 = feedback-in #3(w398) -> ()
            }
            frame #1 {
              n288 = Dequeue Element(queue=w407) -> (element=w406:string)  [unwired: 2 in, 3 out]
              n289 = UDP Write(address=w410, port or service name=w413, connection ID=w412, data in=w406, 8:w411) -> (error out=w408:errorcluster, 3:w409:refnum<k16>)  [unwired: 1 in]
            }
          }
          n290 = local read "stop"() -> (w375:bool)
          n291 = Unbundle(w377) -> ("status"=w378:bool)  [unwired: 2 out]
          n292 = node-c288() -> ()  [unwired: 1 in, 1 out]
          n293 = Compound Arithmetic op=OR(w378, w375) -> (w376:bool)
        }
        n294 = node-c288(w361) -> ()  [unwired: 1 out]
        n295 = UDP Close(connection ID=w368, 8:w366) -> (error out=→"UDP_Out_Error":errorcluster)  [unwired: 1 out]
      }
      n296 = while {
        tunnel: w78 -> [w319]
        tunnel: w79 -> [w318]
        stop <- w322 stop-if-true
        # "TCP Loop writing to SEPTIC Tank"
        n297 = TCP Open Connection(address="192.168.101.108", remote port or service name=u16 3502) -> (connection ID=w325:refnum<k5>, error out=w320:errorcluster)  [unwired: 3 in]
        n298 = case shown="No Error" w320 {
          selector: w320 -> [w330 w357]
          tunnel: w325 -> [w335 w358]
          tunnel: [w334 w358] -> w324
          tunnel: [w333 w357] -> w323
          tunnel: [w332 w356] -> w322
          tunnel: w318 -> [w329 _]
          tunnel: w319 -> [w328 _]
          frame No Error {
            n299 = node-c288() -> (w337:T3)  [unwired: 4 in]
            n300 = timed-loop {
              tunnel: w335 -> [w351]
              tunnel: w330 -> [w350]
              tunnel: [w349] -> w334
              tunnel: [w348] -> w333
              tunnel: [w338] -> w332
              shift-right: [w342] -> _
              shift-left: FALSE -> [w345]
              timing: w337 -> [_]
              timing-out: [_] -> w336
              tunnel: w329 -> [w341]
              tunnel: w328 -> [w340]
              stop <- w346 stop-if-true
              n301 = node-c288() -> ()  [unwired: 1 in, 1 out]
              n302 = Dequeue Element(queue=w341, error in (no error)=w340) -> (element=w339:string)  [unwired: 1 in, 3 out]
              n303 = Select(t=FALSE, s=w345, f=TRUE) -> (s? t:f=w342:bool)
              "TCP packet\nSend to SEPTIC" <- w342
              n304 = TCP Write(connection ID=w351, data in=w339, error in (no error)=w350) -> (connection ID out=w349:refnum<k5>, error out=w348:errorcluster)  [unwired: 1 in, 1 out]
              n305 = local read "stop"() -> (w338:bool)
              n306 = Unbundle(w348) -> ("status"=w347:bool)  [unwired: 2 out]
              n307 = node-c288() -> ()  [unwired: 1 in, 1 out]
              n308 = Compound Arithmetic op=OR(w347, w338) -> (w346:bool)
            }
            n309 = node-c288(w336) -> ()  [unwired: 1 out]
          }
          frame Error {
            n310 = local read "stop"() -> (w356:bool)
          }
        }
        n311 = TCP Close Connection(connection ID=w324, error in (no error)=w323) -> (error out=→"SEPTIC TCP Error Out":errorcluster)  [unwired: 1 in, 1 out]
        n312 = Wait (ms)(milliseconds to wait=u32 1000) -> ()  [unwired: 1 out]
      }
      n313 = while {
        tunnel: w85 -> [w418]
        tunnel: w84 -> [w417]
        stop <- w421 stop-if-true
        # "TCP Loop writing to FISH Tank"
        n314 = TCP Open Connection(address="192.168.101.110", remote port or service name=u16 3502) -> (connection ID=w424:refnum<k5>, error out=w419:errorcluster)  [unwired: 3 in]
        n315 = case shown="No Error" w419 {
          selector: w419 -> [w429 w456]
          tunnel: w424 -> [w434 w457]
          tunnel: [w433 w457] -> w423
          tunnel: [w432 w456] -> w422
          tunnel: [w431 w455] -> w421
          tunnel: w418 -> [w428 _]
          tunnel: w417 -> [w427 _]
          frame No Error {
            n316 = node-c288() -> (w436:T3)  [unwired: 4 in]
            n317 = timed-loop {
              tunnel: w434 -> [w450]
              tunnel: w429 -> [w449]
              tunnel: [w448] -> w433
              tunnel: [w447] -> w432
              tunnel: [w444] -> w431
              shift-right: [w440] -> _
              shift-left: FALSE -> [w443]
              timing: w436 -> [_]
              timing-out: [_] -> w435
              tunnel: w428 -> [w439]
              tunnel: w427 -> [w438]
              stop <- w445 stop-if-true
              n318 = node-c288() -> ()  [unwired: 1 in, 1 out]
              n319 = Dequeue Element(queue=w439, error in (no error)=w438) -> (element=w437:string)  [unwired: 1 in, 3 out]
              n320 = Select(t=FALSE, s=w443, f=TRUE) -> (s? t:f=w440:bool)
              "TCP packet\nSend to FISH" <- w440
              n321 = TCP Write(connection ID=w450, data in=w437, error in (no error)=w449) -> (connection ID out=w448:refnum<k5>, error out=w447:errorcluster)  [unwired: 1 in, 1 out]
              n322 = local read "stop"() -> (w444:bool)
              n323 = Unbundle(w447) -> ("status"=w446:bool)  [unwired: 2 out]
              n324 = node-c288() -> ()  [unwired: 1 in, 1 out]
              n325 = Compound Arithmetic op=OR(w446, w444) -> (w445:bool)
            }
            n326 = node-c288(w435) -> ()  [unwired: 1 out]
          }
          frame Error {
            n327 = local read "stop"() -> (w455:bool)
          }
        }
        n328 = TCP Close Connection(connection ID=w423, error in (no error)=w422) -> (error out=→"FISH TCP Error Out":errorcluster)  [unwired: 1 in, 1 out]
        n329 = Wait (ms)(milliseconds to wait=u32 1000) -> ()  [unwired: 1 out]
      }
      n330 = node-c288(w63) -> ()  [unwired: 1 out]
    }
    frame Error {
    }
  }
  n331 = VISA Close(VISA resource name=w36, error in (no error)=w35) -> (error out=→"Serial Visa Error":errorcluster)
